vi "PXI-Init Channel Array.vi"(0 "Sorted channel names":string[](array[string])=["AI01", "AI02", "AI03", "AI04", "AI05", "AI06", "AI07", "AI08", "AI09", "AI10", "AI11", "AI12", "AI13", "AI14", "AI15", "AI16", "AI17", "AI18", "AI19", "AI20", "AI21", "AI22", "AO01", "AO02", "AO03", "AO04", "AO05", "AO06", "AO07", "AO08", "AO09", "AO10"], 5 "Sorted physical channels":tag[](array[tag]), 11 "error in (no error)":errorcluster) -> (4 "Channel Array":T1[](array[typedef]) {"Terminal configuration" items=["Default"=-1, "RSE"=10083, "Differential"=10106, "Pseudodifferential"=12529]}, 15 "error out":errorcluster)   [LabVIEW 2020]
uses:
  Type Defs/Channel Struct.ctl
  PXI Globals.vi
panel:
  in  "Dummy Channel struct":T1={"Channel name"="AI1", "Vmax"=10.0, "Vmin"=204800.0, "Rate"=-1.0, "Terminal configuration"=10, "Physical Channel"="", "Regenerate"=FALSE} {"Terminal configuration" items=["Default"=-1, "RSE"=10083, "Differential"=10106, "Pseudodifferential"=12529]}
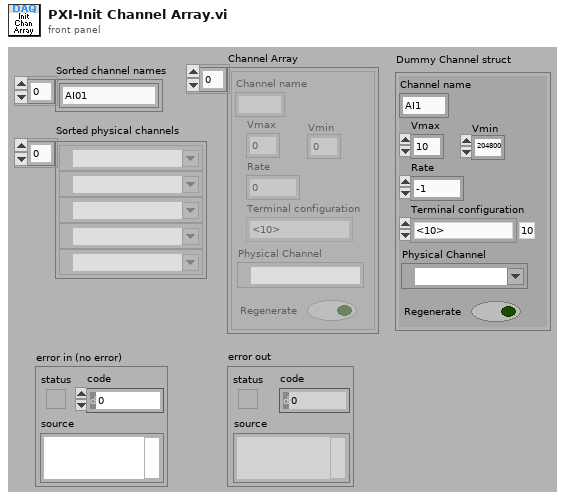
[diagram p1: front panel]
types:
  T1 = typedef "Channel Struct.ctl" = cluster{"Channel name":string, "Vmax":dbl, "Vmin":dbl, "Rate":dbl, "Terminal configuration":i32, "Physical Channel":tag, "Regenerate":bool}
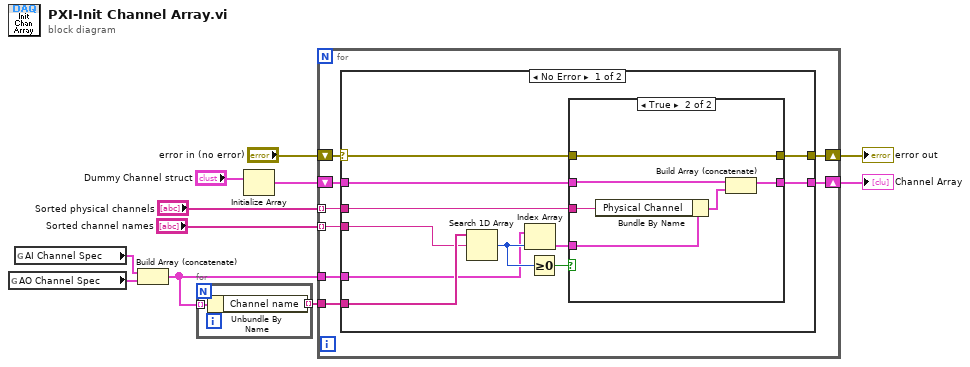
[diagram p0: block diagram]
diagram:
  n1 = global read "PXI Globals.vi" "AO Channel Spec"() -> (w7:T1[])
  n2 = global read "PXI Globals.vi" "AI Channel Spec"() -> (w8:T1[])
  n3 = Build Array (concatenate)(w8, w7) -> (w2:T1[])
  n4 = for {
    tunnel: w2 -> [w13] mode=indexing
    tunnel: [w12] -> w1 mode=indexing
    n5 = Unbundle By Name(w13) -> ("Channel name"=w12:string)
  }
  n6 = Initialize Array("Dummy Channel struct") -> (w10:T1[])  [unwired: 1 in]
  n7 = for {
    shift-right: [w20] -> w9
    shift-left: w10 -> [w21]
    tunnel: w2 -> [w18]
    tunnel: "Sorted channel names" -> [w19] mode=indexing
    tunnel: "Sorted physical channels" -> [w17] mode=indexing
    shift-right: [w16] -> w4
    shift-left: "error in (no error)" -> [w15]
    tunnel: w1 -> [w14]
    n8 = case shown="No Error" w15 {
      selector: w15 -> [w26 w42]
      tunnel: w21 -> [w32 w41]
      tunnel: [w31 w41] -> w20
      tunnel: w19 -> [w24 _]
      tunnel: w18 -> [w23 _]
      tunnel: w17 -> [w22 _]
      tunnel: [w27 w42] -> w16
      tunnel: w14 -> [w25 _]
      frame No Error {
        n9 = Search 1D Array(1D array=w25, element=w24) -> (index of element=w29:i32)  [unwired: 1 in]
        n10 = Index Array(array=w23, index=w29) -> (element=w28:T1)
        n11 = Greater Or Equal To 0?(x=w29) -> (x >= 0?=w30:bool)
        n12 = case shown="True" w30 {
          tunnel: w32 -> [w34 w37]
          tunnel: [w34 w35] -> w31
          tunnel: w28 -> [_ w38]
          tunnel: [w33 w40] -> w27
          tunnel: w26 -> [w33 w40]
          tunnel: w22 -> [_ w39]
          frame False {
          }
          frame True {
            n13 = Bundle By Name(cluster=w38, "Physical Channel"=w39) -> (w36:T1)
            n14 = Build Array (concatenate)(w37, w36) -> (w35:T1[])
          }
        }
      }
      frame Error {
      }
    }
  }
  "Channel Array" <- w9
  "error out" <- w4
